vi "List Directory__ogtk.vi"(4 "error in (no error)":errorcluster, 6 "pattern":string, 7 "directory path":path) -> (0 "error out":errorcluster, 1 "directory names":string[](array[string]), 2 "file names":string[](array[string]), 3 "dup directory path":path)   [LabVIEW 2020]
doc: "Augments the primitive List Directory function by allowing multiple semicolon delimited patterns."
uses:
  Trim Whitespace (String)__ogtk.vi
  <userlib>/_OpenG.lib/array/array.llb/Remove Duplicates from 1D Array (String)__ogtk.vi
panel:
  # "[OpenG VI Tags] ***Do Not Remove***"
  # "List Directory.vi - Augments the primitive List Directory function by\nallowing semicolon delimited patterns.\n\nCopyright (C) 2002 James Kring jim@jimkring.com\n\nPlease visit http://www.OpenG.org to learn about the\nOpen Source LabVIEW software movement.\n\nThis library is free software; you can redistribute it and/or\nmodify it under the terms of the GNU Lesser General Public\nLicense as published by the Free Software Foundation; either\nversion 2.1 of the License, or (at your option) any later version.\nThis library is distributed in the hope that it will be useful,\nbut WITHOUT ANY WARRANTY; without even the implied warranty of\nMERCHANTABILITY or FITNESS FOR A PARTICULAR PURPOSE. See the GNU\nLesser General Public License for more details.\nYou should have received a copy of the GNU Lesser General Public\nLicense along with this library; if not, write to the Free Software\nFoundation, Inc., 59 Temple Place, Suite 330, Boston, MA 02111-1307 USA"
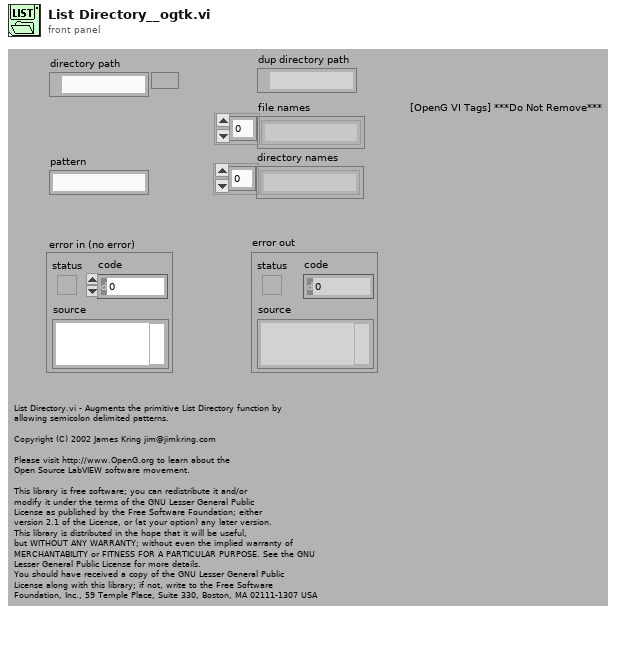
[diagram p1: front panel]
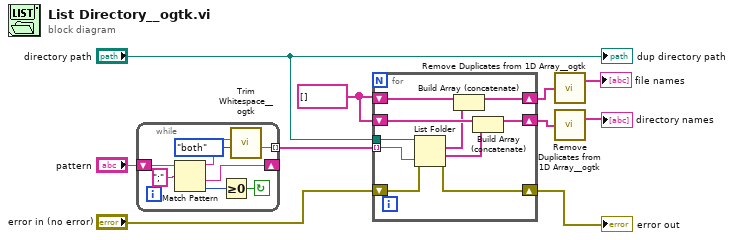
[diagram p0: block diagram]
diagram:
  w5 = string[] [] ("file names")
  n1 = while {
    shift-right: [w18] -> _
    shift-left: "pattern" -> [w15]
    tunnel: [w12] -> w10 mode=indexing
    stop <- w17 continue-if-true
    n2 = Match Pattern(string=w15, regular expression=";" ("pattern")) -> (before substring=w14:string, after substring=w18:string, offset past match=w16:i32)  [unwired: 1 in, 1 out]
    n3 = Greater Or Equal To 0?(x=w16) -> (x >= 0?=w17:bool)
    n4 = call-poly "Trim Whitespace__ogtk.vi"("Remove (leading and trailing)"=enum16{"leading", "trailing", "both"}."both" ("remove (leading and trailing)"), "String in"=w14) -> ("String out"=w12:string)  [unwired: 5 in]
  }
  n5 = for {
    tunnel: w10 -> [w28] mode=indexing
    shift-right: [w26] -> w8
    shift-left: "error in (no error)" -> [w27]
    tunnel: "directory path" -> [w25]
    shift-right: [w23] -> w2
    shift-left: w5 -> [w24]
    shift-right: [w21] -> w4
    shift-left: w5 -> [w22]
    n6 = List Folder(path=w25, pattern=w28, error in=w27) -> (filenames=w19:string[], folder names=w20:string[], error out=w26:errorcluster)  [unwired: 1 in, 1 out]
    n7 = Build Array (concatenate)(w24, w19) -> (w23:string[])
    n8 = Build Array (concatenate)(w22, w20) -> (w21:string[])
  }
  "error out" <- w8
  n9 = call-poly <userlib>:"Remove Duplicates from 1D Array__ogtk.vi"("Input Array"=w2) -> ("Output Array"=→"file names":string[])  [unwired: 1 out]
  n10 = call-poly <userlib>:"Remove Duplicates from 1D Array__ogtk.vi"("Input Array"=w4) -> ("Output Array"=→"directory names":string[])  [unwired: 1 out]
  "dup directory path" <- "directory path"
